vi "SIAM-convertReturnToReadable.vi"(8 "error in (no error)":errorcluster, 11 "Return":i32[](array[numeric]) format="%.0x") -> (0 "error out":errorcluster, 2 "CR?":string, 3 "Readable":string)   [LabVIEW 2011]
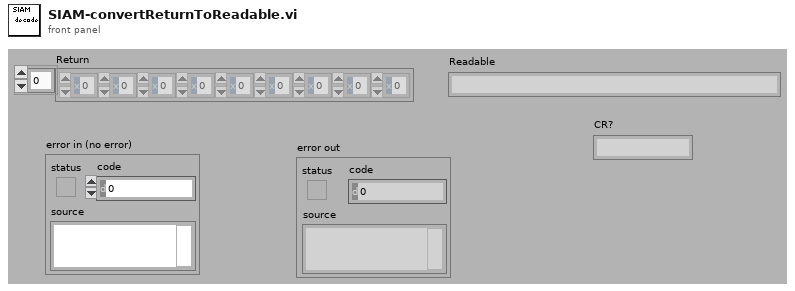
[diagram p1: front panel]
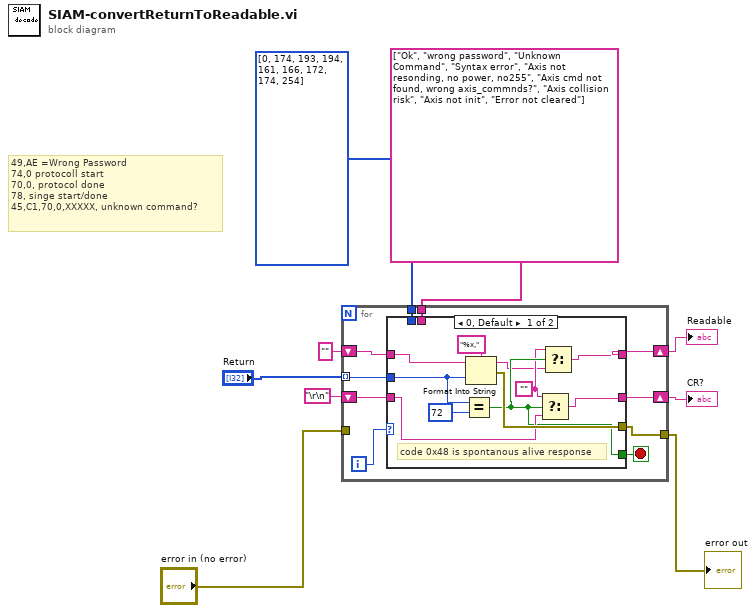
[diagram p0: block diagram]
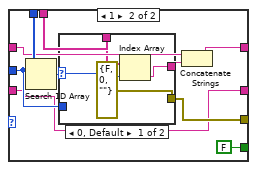
[diagram p2: hidden frame]
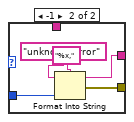
[diagram p3: hidden frame]
diagram:
  # "49,AE =Wrong Password\n74,0 protocoll start\n70,0, protocol done\n78, singe start/done\n45,C1,70,0,XXXXX, unknown command?"
  n1 = for {
    tunnel: "Return" -> [w19] mode=indexing
    shift-right: [w17] -> w9
    shift-left: "" -> [w18]
    tunnel: u32[] [0, 174, 193, 194, 161, 166, 172, 174, 254] -> [w15]
    tunnel: string[] ["Ok", "wrong password", "Unknown Command", "Syntax error", "Axis not resonding, no power, no255", "Axis cmd not found, wrong axis_commnds?", "Axis collision risk", "Axis not init", "Error not cleared"] ("Array") -> [w14]
    tunnel: "error in (no error)" -> [_]
    tunnel: [w13] -> w3
    shift-right: [w12] -> w2
    shift-left: "\r\n" -> [w11]
    i -> [w16]
    stop <- w10 stop-if-true
    n2 = case shown="0, Default" w16 {
      tunnel: w19 -> [w27 w34]
      tunnel: w18 -> [w29 w39]
      tunnel: [w20 w37] -> w17
      tunnel: w15 -> [_ w40]
      tunnel: w14 -> [_ w38]
      tunnel: [w28 w33] -> w13
      tunnel: [w24 w32] -> w12
      tunnel: w11 -> [w25 w32]
      tunnel: [w23 FALSE] -> w10
      frame 0, Default {
        w22 = ""
        # "code 0x48 is spontanous alive response"
        n3 = Equal?(x=w27, y=72) -> (x = y?=w23:bool)
        n4 = Format Into String(format string="%x,", initial string=w29, w27) -> (resulting string=w21:string, error out=w28:errorcluster)  [unwired: 1 in]
        n5 = Select(t=w22, s=w23, f=w25) -> (s? t:f=w24:string)
        n6 = Select(t=w22, s=w23, f=w21) -> (s? t:f=w20:string)
      }
      frame 1 {
        n7 = Search 1D Array(1D array=w40, element=w34) -> (index of element=w35:i32)  [unwired: 1 in]
        n8 = case shown="0, Default" w35 {
          selector: w35 -> [w42 _]
          tunnel: w38 -> [w44 _]
          tunnel: [w43 w46] -> w36
          tunnel: w34 -> [_ w49]
          tunnel: [errorcluster {"status"=FALSE, "code"=0, "source"=""} ("error IO") w45] -> w33
          frame 0, Default {
            n9 = Index Array(array=w44, index=w42) -> (element=w43:string)
          }
          frame -1 {
            n10 = Format Into String(format string="%x,", initial string="unknown error", w49) -> (resulting string=w46:string, error out=w45:errorcluster)  [unwired: 1 in]
          }
        }
        n11 = Concatenate Strings(w39, w36) -> (w37:string)
      }
    }
  }
  "Readable" <- w9
  "error out" <- w3
  "CR?" <- w2
